vi "Save Load Accuracy Data.vi"(6 "Total AD Counts":dbl[][](array[numeric]), 7 "Shim #":i32, 8 "error in (no error)":errorcluster, 9 "Avg AD Counts":dbl[][](array[numeric]), 10 "AD Counts":dbl[][](array[numeric]), 11 "LA Cycle #":i32) -> (0 "error out":errorcluster, 1 "NFHU Error Code":i32, 2 "Error Code":i32, 3 "Pass?":bool, 5 "NFHU Pass?":bool)   [LabVIEW 2015]
uses:
  <vilib>/addons/_office/excel.llb/Excel Easy Table (num).vi
  <vilib>/Utility/NIReport.llb/NI_report.lvclass
  <vilib>/addons/_office/NI_ReportGenerationToolkit.lvlib
  <vilib>/Utility/NIReport.llb/Excel/NI_Excel.lvclass
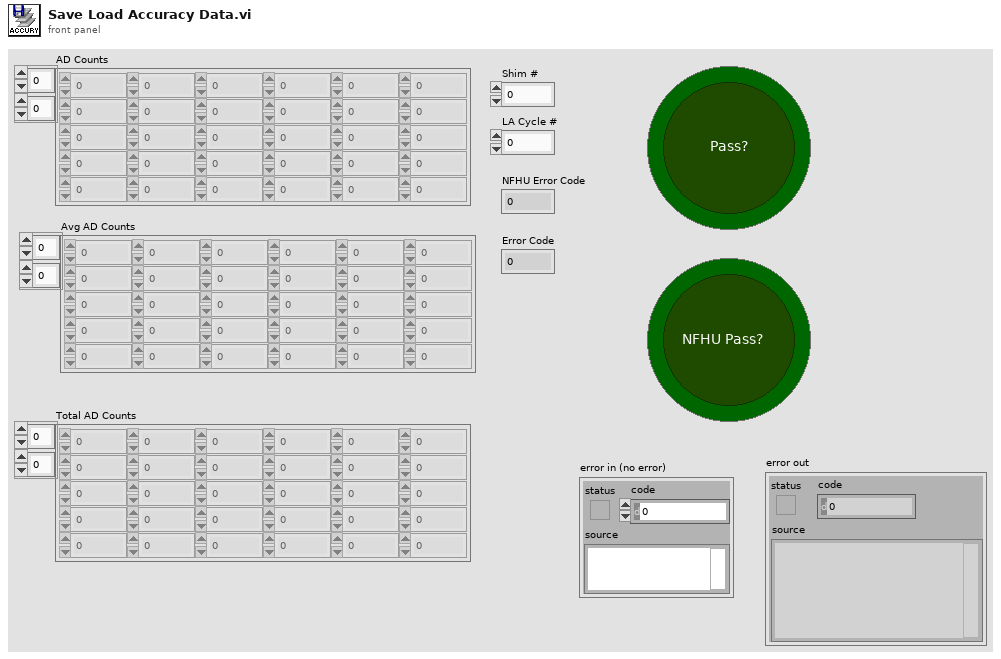
[diagram p1: front panel]
types:
  T1 = enum16{"maximized", "minimized", "normal", "no change"}
  T2 = enum16{"Standard Report", "HTML", "Word", "Excel"}
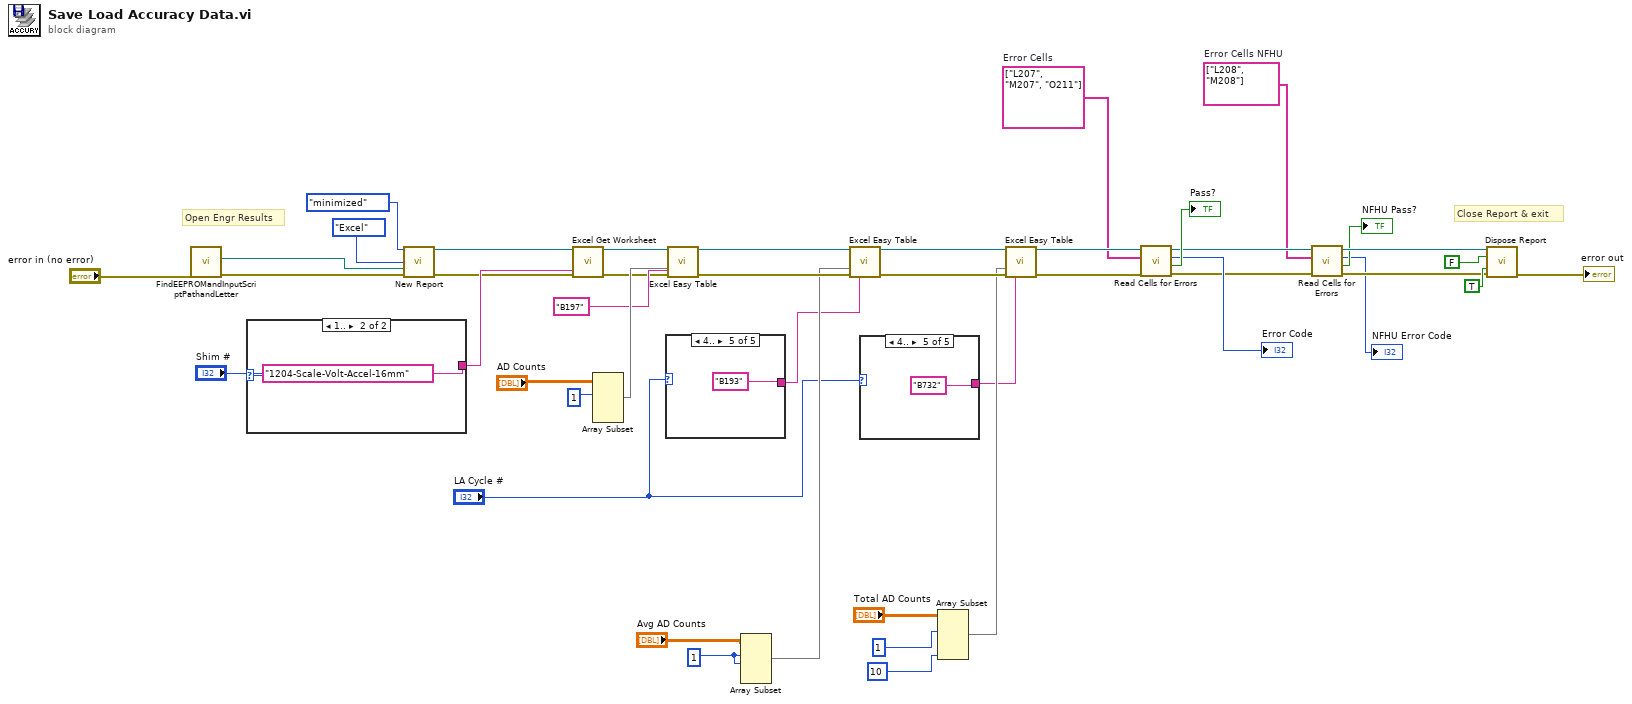
[diagram p0: block diagram]
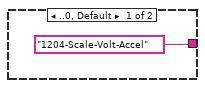
[diagram p2: hidden frame]
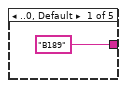
[diagram p3: hidden frame]
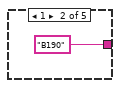
[diagram p4: hidden frame]
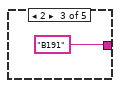
[diagram p5: hidden frame]
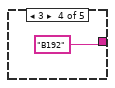
[diagram p6: hidden frame]
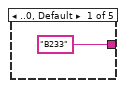
[diagram p7: hidden frame]
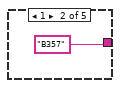
[diagram p8: hidden frame]
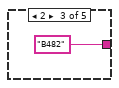
[diagram p9: hidden frame]
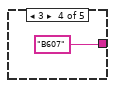
[diagram p10: hidden frame]
diagram:
  w1 = string[] ["L208", "M208"]  # Error Cells NFHU
  w2 = string[] ["L207", "M207", "O211"]  # Error Cells
  w15 = 1 ("length")
  # "Close Report & exit"
  # "Open Engr Results"
  n1 = call "FindEEPROMandInputScriptPathandLetter.vi"("Error In"="error in (no error)") -> ("Error Out"=w35:errorcluster, "Engr Result Path"=w44:path)  [unwired: 6 in, 1 out]
  n2 = case shown="1.." "Shim #" {
    tunnel: ["1204-Scale-Volt-Accel" ("name (\"\")") "1204-Scale-Volt-Accel-16mm" ("name (\"\")")] -> w41
    frame ..0, Default {
    }
    frame 1.. {
    }
  }
  n3 = call <vilib>:"New Report.vi"("window state (normal)"=T1."minimized", "report type"=T2."Excel", "template (empty)"=w44, "error in (no error)"=w35) -> ("report out"=w38:refnum<class "NI_report.lvclass">, "error out"=w37:errorcluster)  [unwired: 10 in]
  n4 = call <vilib>:"Excel Get Worksheet.vi"("report in"=w38, "error in (no error)"=w37, "name (\"\")"=w41) -> ("report out"=w27:refnum<class "NI_report.lvclass">, "error out"=w26:errorcluster)  [unwired: 11 in]
  n5 = Array Subset(array="AD Counts", index (row)=1 ("length")) -> (w29:dbl[][])  [unwired: 3 in]
  n6 = case shown="4.." "LA Cycle #" {
    tunnel: ["B189" ("name (\"\")") "B190" ("name (\"\")") "B191" ("name (\"\")") "B192" ("name (\"\")") "B193" ("name (\"\")")] -> w5
    frame ..0, Default {
    }
    frame 1 {
    }
    frame 2 {
    }
    frame 3 {
    }
    frame 4.. {
    }
  }
  n7 = call-poly <vilib>:"Excel Easy Table.vi"("report in"=w27, "text data"=w29, "error in (no error)"=w26, "name (\"\")"="B197" ("name (\"\")")) -> ("report out"=w19:refnum<class "NI_report.lvclass">, "error out"=w18:errorcluster)  [unwired: 7 in, 3 out]
  n8 = Array Subset(array="Avg AD Counts", index (row)=w15, length (row)=w15) -> (w16:dbl[][])  [unwired: 2 in]
  n9 = call-poly <vilib>:"Excel Easy Table.vi"("report in"=w19, "text data"=w16, "error in (no error)"=w18, "name (\"\")"=w5) -> ("report out"=w14:refnum<class "NI_report.lvclass">, "error out"=w12:errorcluster)  [unwired: 7 in, 3 out]
  n10 = case shown="4.." "LA Cycle #" {
    tunnel: ["B233" ("name (\"\")") "B357" ("name (\"\")") "B482" ("name (\"\")") "B607" ("name (\"\")") "B732" ("name (\"\")")] -> w6
    frame ..0, Default {
    }
    frame 1 {
    }
    frame 2 {
    }
    frame 3 {
    }
    frame 4.. {
    }
  }
  n11 = Array Subset(array="Total AD Counts", index (row)=1 ("length"), length (col)=10 ("length")) -> (w7:dbl[][])  [unwired: 2 in]
  n12 = call-poly <vilib>:"Excel Easy Table.vi"("report in"=w14, "text data"=w7, "error in (no error)"=w12, "name (\"\")"=w6) -> ("report out"=w13:refnum<class "NI_report.lvclass">, "error out"=w11:errorcluster)  [unwired: 7 in, 3 out]
  n13 = call "Read Cells for Errors.vi"("error in (no error)"=w11, "Error Cells (ex:A12)"=w2, "NI_report in"=w13) -> ("error out"=w25:errorcluster, "Pass?"=→"Pass?":bool, "Error Code"=→"Error Code":i32, "NI_report out"=w23:refnum<class "NI_report.lvclass">)  [unwired: 5 in]
  n14 = call "Read Cells for Errors.vi"("error in (no error)"=w25, "Error Cells (ex:A12)"=w1, "NI_report in"=w23) -> ("error out"=w24:errorcluster, "Pass?"=→"NFHU Pass?":bool, "Error Code"=→"NFHU Error Code":i32, "NI_report out"=w22:refnum<class "NI_report.lvclass">)  [unwired: 5 in]
  n15 = call-dynamic "Dispose Report.vi"("report in"=w22, "wait until printing completed? (T)"=FALSE, "save changes? (F)"=TRUE, "error in (no error)"=w24) -> ("error out"=→"error out":errorcluster)  [unwired: 11 in]
